vi "Write Device(s)Settings.vi"(8 "error in (no error)":errorcluster, 10 "Device(s)Settings":T1 {"Phase Select" items=["Phase ALL", "Phase A", "Phase B", "Phase C"]}, 11 "NHRDCPower in":refnum<class "NHRDCPower.lvclass">) -> (0 "error out":errorcluster, 3 "NHRDCPower out":refnum<class "NHRDCPower.lvclass">)   [LabVIEW 2018, in "AcPwrPlugins.lvlib" / "NHRDCPower.lvclass"]
uses:
  NHRDCPower.lvclass
  TypeDefs/Device(s)Settings.ctl
  NHRDCPower.lvclass/NHRDCPower.ctl
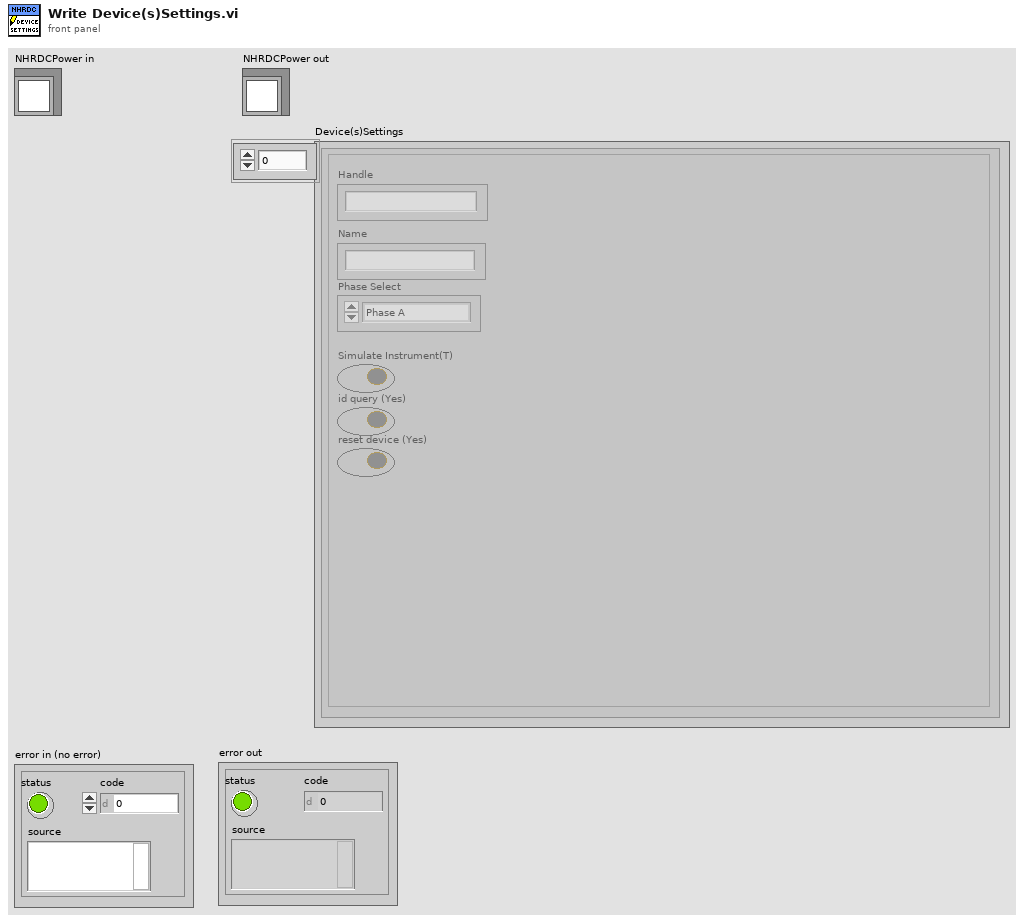
[diagram p1: front panel]
types:
  T1 = typedef "AcPwrPlugins.lvlib/NHRDCPower.lvclass/Device(s)Settings.ctl" = cluster{"Handle":string, "Name":string, "Phase Select":i32, "id query (Yes)":bool, "reset device (Yes)":bool, "Connected":bool, "Voltage Range (V)":dbl[], "Timing":cluster{"TimingOn":enum16{""}, "Hours":u32, "Minutes":u32, "Seconds":dbl, "CutoffVoltage":dbl}, "Simulate Instrument(T)":bool}[]
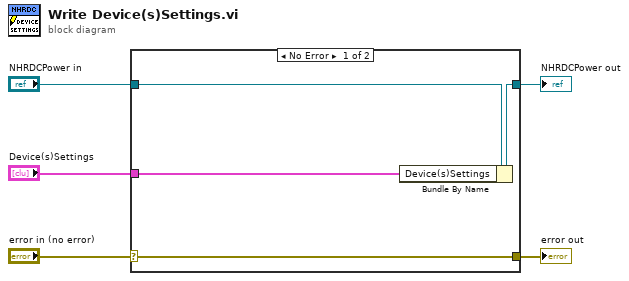
[diagram p0: block diagram]
diagram:
  n1 = case shown="No Error" "error in (no error)" {
    selector: "error in (no error)" -> [w9 w10]
    tunnel: [w9 w10] -> w4
    tunnel: [w7 w11] -> w2
    tunnel: "NHRDCPower in" -> [w8 w11]
    tunnel: "Device(s)Settings" -> [w6 _]
    frame No Error {
      n2 = Bundle By Name(cluster=w8, "Device(s)Settings"=w6) -> (w7:refnum<class "NHRDCPower.lvclass">)
    }
    frame Error {
    }
  }
  "error out" <- w4
  "NHRDCPower out" <- w2
